vi "Sort Complex Numbers (Mag and Phase).vi"(10 "Order":enum16{"Ascending", "Descending"}(ring), 11 "Complex Numbers":cdb[](array[numeric])) -> (0 "error":i32, 2 "Sorted Index":i32[](array[numeric]), 3 "Sorted Complex Numbers":cdb[](array[numeric]))   [LabVIEW 2014, in "NI_AALPro.lvlib"]
uses:
  NI_AALPro.lvlib
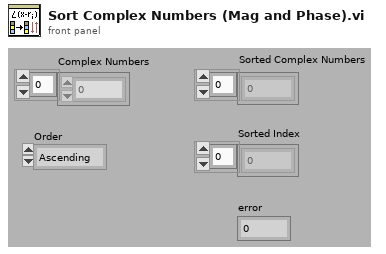
[diagram p1: front panel]
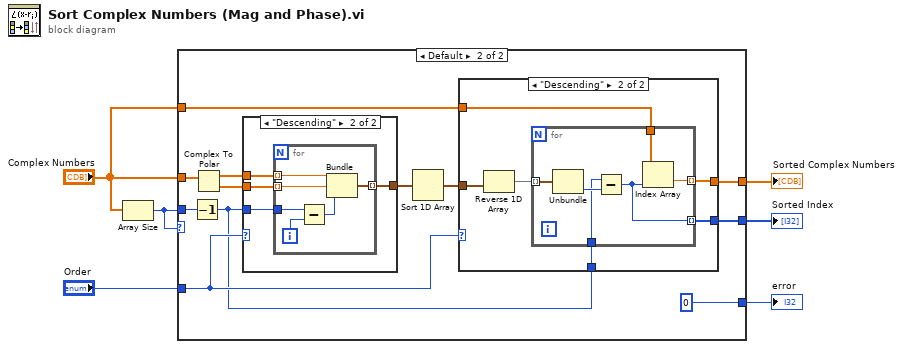
[diagram p0: block diagram]
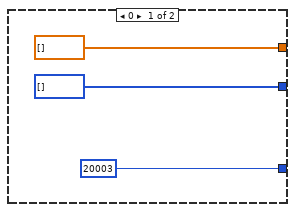
[diagram p2: hidden frame]
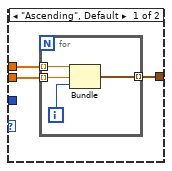
[diagram p3: hidden frame]
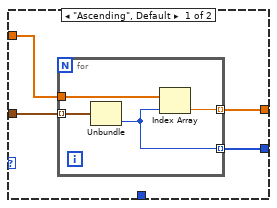
[diagram p4: hidden frame]
diagram:
  n1 = Array Size(array="Complex Numbers") -> (size(s)=w2:i32)
  n2 = case shown="Default" w2 {
    tunnel: "Complex Numbers" -> [_ w18]
    tunnel: [cdb[] [] ("CDB") w13] -> w6
    tunnel: [i32[] [] w12] -> w5
    tunnel: "Order" -> [_ w15]
    tunnel: [20003 ("empty array") 0] -> w3
    tunnel: w2 -> [_ w14]
    tunnel: "Complex Numbers" -> [_ w11]
    frame 0 {
    }
    frame Default {
      n3 = Decrement(x=w14) -> (x-1=w10:i32)
      n4 = Complex To Polar(r * e^(i*theta)=w18) -> (r=w20:dbl[], theta=w19:dbl[])
      n5 = case shown="\"Descending\"" w15 {
        tunnel: [w24 w32] -> w21
        tunnel: w20 -> [w23 w31]
        tunnel: w19 -> [w22 w30]
        tunnel: w10 -> [_ w29]
        frame "Ascending", Default {
          n6 = for {
            tunnel: w23 -> [w28] mode=indexing
            tunnel: w22 -> [w26] mode=indexing
            tunnel: [w27] -> w24 mode=indexing
            i -> [w25]
            n7 = Bundle("Numeric"=w28, "Numeric"=w26, w25) -> (w27:cluster{"Numeric":dbl, "Numeric":dbl, i32})  [unwired: 1 in]
          }
        }
        frame "Descending" {
          n8 = for {
            tunnel: w31 -> [w38] mode=indexing
            tunnel: w30 -> [w36] mode=indexing
            tunnel: [w37] -> w32 mode=indexing
            tunnel: w29 -> [w34]
            i -> [w35]
            n9 = Subtract(x=w34, y=w35) -> (x-y=w33:i32)
            n10 = Bundle("Numeric"=w38, "Numeric"=w36, w33) -> (w37:cluster{"Numeric":dbl, "Numeric":dbl, i32})  [unwired: 1 in]
          }
        }
      }
      n11 = Sort 1D Array(array=w21) -> (sorted array=w17:cluster{"Numeric":dbl, "Numeric":dbl, i32}[])
      n12 = case shown="\"Descending\"" w15 {
        tunnel: w17 -> [w42 w52]
        tunnel: [w41 w50] -> w13
        tunnel: [w40 w48] -> w12
        tunnel: w11 -> [w39 w47]
        tunnel: w10 -> [_ w49]
        frame "Ascending", Default {
          n13 = for {
            tunnel: w42 -> [w46] mode=indexing
            tunnel: [w44] -> w41 mode=indexing
            tunnel: [w43] -> w40 mode=indexing
            tunnel: w39 -> [w45]
            n14 = Unbundle(w46) -> (w43:i32)  [unwired: 2 out]
            n15 = Index Array(array=w45, index=w43) -> (element=w44:cdb)
          }
        }
        frame "Descending" {
          n16 = Reverse 1D Array(array=w52) -> (reversed array=w51:cluster{"Numeric":dbl, "Numeric":dbl, i32}[])
          n17 = for {
            tunnel: w51 -> [w58] mode=indexing
            tunnel: [w54] -> w50 mode=indexing
            tunnel: w49 -> [w56]
            tunnel: [w55] -> w48 mode=indexing
            tunnel: w47 -> [w53]
            n18 = Unbundle(w58) -> (w57:i32)  [unwired: 2 out]
            n19 = Subtract(x=w56, y=w57) -> (x-y=w55:i32)
            n20 = Index Array(array=w53, index=w55) -> (element=w54:cdb)
          }
        }
      }
    }
  }
  "Sorted Complex Numbers" <- w6
  "Sorted Index" <- w5
  "error" <- w3
